vi "Read Plugin State Data.vi"(8 "error in (no error)":errorcluster, 10 "plugin index":i32, 11 "Framework Status in":refnum<class "Framework Status.lvclass">) -> (0 "error out":errorcluster, 1 "groups state data":T1[](array[typedef]) {"duration" format="%d us"}, 2 "plugin state data":T1 {"duration" format="%d us"}, 3 "Framework Status out":refnum<class "Framework Status.lvclass">)   [LabVIEW 2017, in "DSF Core.lvlib" / "Framework Status.lvclass"]
uses:
  Framework Status.lvclass
  Status/Status Data.ctl
  Status/Status Pointer.lvclass
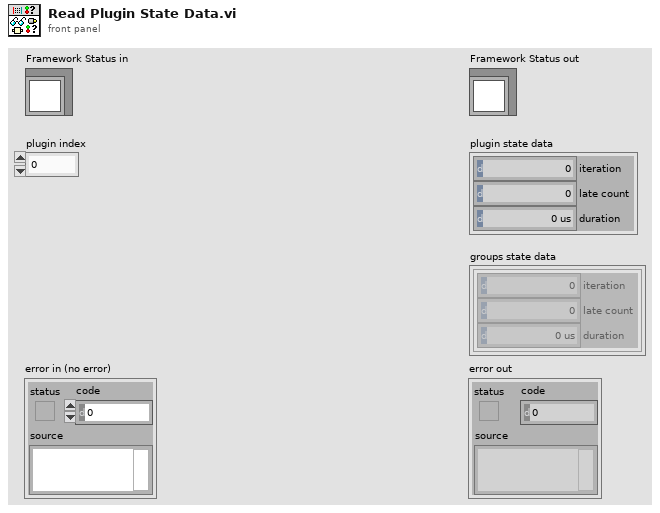
[diagram p1: front panel]
types:
  T1 = typedef "DSF Core.lvlib/Status Pointer.lvclass/Status Data.ctl" = cluster{"iteration":u64, "late count":i32, "duration":u32}
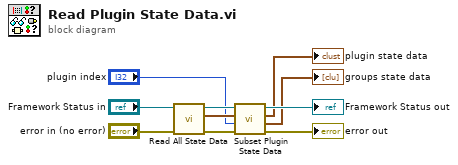
[diagram p0: block diagram]
diagram:
  n1 = call "Read All State Data.vi"("error in (no error)"="error in (no error)", "Framework Status in"="Framework Status in") -> ("error out"=w7:errorcluster, "all state data"=w8:T1[], "Framework Status out"=w6:refnum<class "Framework Status.lvclass">)  [unwired: 7 in]
  n2 = call "Subset Plugin State Data.vi"("error in (no error)"=w7, "plugin index"="plugin index", "all state data"=w8, "Framework Status in"=w6) -> ("error out"=→"error out":errorcluster, "groups state data"=→"groups state data":T1[], "plugin state data"=→"plugin state data":T1, "Framework Status out"=→"Framework Status out":refnum<class "Framework Status.lvclass">)  [unwired: 4 in]
